vi "Balance Inquiry.vi"(8 "error in (no error)":errorcluster, 11 "ATM Controller in":refnum<class "ATM Controller.lvclass">) -> (0 "error out":errorcluster, 3 "ATM Controller out":refnum<class "ATM Controller.lvclass">)   [LabVIEW 2020, in "ATM Controller.lvclass"]
uses:
  ATM Controller.lvclass
  State.ctl
  ATM Controller.lvclass/ATM Controller.ctl
  Account Database/Account Database.lvclass
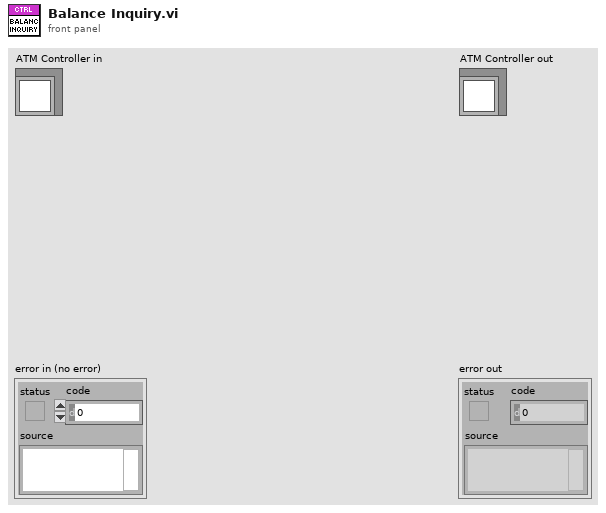
[diagram p1: front panel]
types:
  T1 = typedef "ATM Controller.lvclass/State.ctl" = enum16{"Start", "Card Inserted", "Verification Failed", "Verification Succeeded", "Depositing", "Depositing Completed", "Withdrawing", "Withdraw Completed", "Withdraw Failed", "Balance Inquiry", "Terminate"}
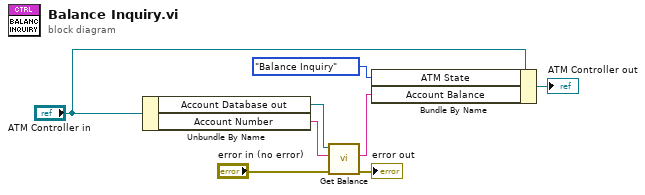
[diagram p0: block diagram]
diagram:
  n1 = Unbundle By Name("ATM Controller in") -> ("Account Database out"=w5:refnum<class "Account Database.lvclass">, "Account Number"=w6:string)
  n2 = call "Get Balance.vi"("error in (no error)"="error in (no error)", "Account Number"=w6, "Account Database in"=w5) -> ("error out"=→"error out":errorcluster, "Account Balance"=w3:string)  [unwired: 6 in, 1 out]
  n3 = Bundle By Name(cluster="ATM Controller in", "ATM State"=State."Balance Inquiry", "Account Balance"=w3) -> (→"ATM Controller out":refnum<class "ATM Controller.lvclass">)
